vi "06_1.vi"() -> ()   [LabVIEW 2018]
uses:
  <userlib>/_OpenG.lib/array/array.llb/Remove Duplicates from 1D Array (U8)__ogtk.vi
panel:
  out "sum":i32
  in  "String":string="wzaopvscxknyjtiul\nbelforsgdhuvmwc\n\nkiocpzjhsetqnwbl\nmaciywlbpodgevujnsktrz\nkpebjfchtlsonwiz\npcezwjtsinxlobk\n\nlrcp\ncdlbepr\nrlqcyutp\nlcpr\nlrtcpym\n\ngxcqbowaelfjhpknz\ngflhackzwqxojeb\nlfwocexqbkjhgaz\n\nfpivaozqnkextmbrjhycdwug\nmotgcrzaisqlpdwbeyhukf\nhbiqcdmkpawueyztgfor\nzrcehkqyoblmtgfiaupdw\n\numjz\njzu\nvzowkpuj\njmzau\n\nunzlx\nlnzxu\nmxluzn\nnzuxli\n\nszkiauhyntdrbcljomqwepv\namowcpzbyukihsjtqelnd\nlzctuqjabmsynphkewxido\nsikblhptcoqemdanywzju\njdeiylutspabcwngfzqkhom\n\nzgyhwtnxjdqucbp\nptnzhudjbcxgkqf\nzgqhjbdnutcmpx\ngjbzhpdxanqcut\n\nwjkcsqlu\nucsjq\n\nvkzsqtunmr\nljcexadhg\n\nfhtrusba\nsvtk\npgzwytn\nastb\n\nhvzjiwlsmnatbxg..."
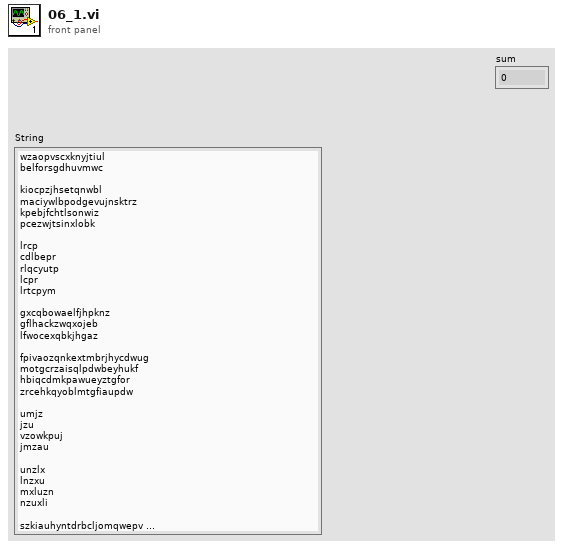
[diagram p1: front panel]
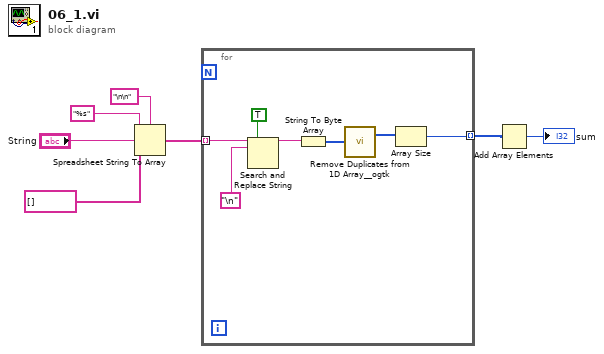
[diagram p0: block diagram]
diagram:
  n1 = Spreadsheet String To Array(delimiter (Tab)="\n\n", format string="%s", spreadsheet string="String", array type (2D Dbl)=string[] []) -> (array=w3:string[])
  n2 = for {
    tunnel: w3 -> [w14] mode=indexing
    tunnel: [w8] -> w2 mode=indexing
    n3 = Search and Replace String(replace all?=TRUE, input string=w14, search string="\n") -> (result string=w11:string)  [unwired: 5 in, 3 out]
    n4 = String To Byte Array(string=w11) -> (unsigned byte array=w10:u8[])
    n5 = call-poly <userlib>:"Remove Duplicates from 1D Array__ogtk.vi"("Input Array"=w10) -> ("Output Array"=w9:u8[])  [unwired: 1 out]
    n6 = Array Size(array=w9) -> (size(s)=w8:i32)
  }
  n7 = Add Array Elements(numeric array=w2) -> (sum=→"sum":i32)
